vi "filter out.vi"(10 "in":dbl[](array[numeric])) -> (2 "out":dbl[](array[numeric]))   [LabVIEW 2010]
uses:
  <vilib>/Analysis/NI_AALBase.lvlib
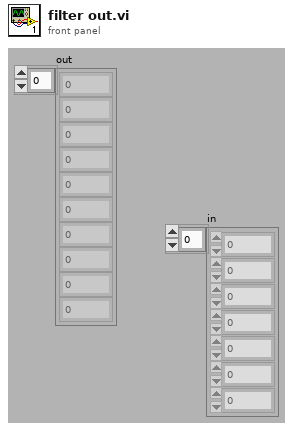
[diagram p1: front panel]
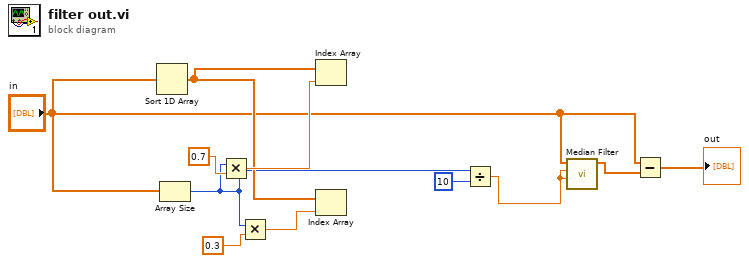
[diagram p0: block diagram]
diagram:
  n1 = Sort 1D Array(array="in") -> (sorted array=w8:dbl[])
  n2 = Array Size(array="in") -> (size(s)=w3:i32)
  n3 = Multiply(x=w3, y=0.7) -> (x*y=w9:dbl)
  n4 = Multiply(x=w3, y=0.3) -> (x*y=w6:dbl)
  n5 = Index Array(array=w8, index=w9) -> ()  [unwired: 1 out]
  n6 = Index Array(array=w8, index=w6) -> ()  [unwired: 1 out]
  n7 = Divide(x=w3, y=10) -> (x/y=w1:dbl)
  n8 = call <vilib>:"Median Filter.vi"("right rank"=w1, "left rank"=w1, "X"="in") -> ("Filtered X"=w11:dbl[])  [unwired: 7 in, 1 out]
  n9 = Subtract(x="in", y=w11) -> (x-y=→"out":dbl[])
